vi "Utility Write To Register - Float or Int.vi"(0 "VISA resource name":refnum<visa-resource-name>, 1 "Unit Address (1)":u8=1, 5 "Register Address (0)":u16, 9 "Data (0)":sgl, 11 "error in (no error)":errorcluster) -> (4 "VISA resource name out":refnum<visa-resource-name>, 15 "error out":errorcluster {"code" format="%.0x"})   [LabVIEW 2010, in "Eurotherm 32xx Series.lvlib"]
doc: "This VI writes the value to the specified register of specified unit."
uses:
  <instrlib>/Eurotherm 32xx Series/Eurotherm 32xx Series.lvlib
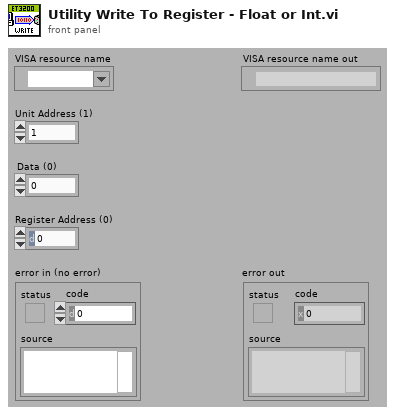
[diagram p1: front panel]
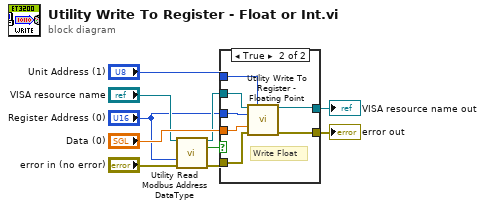
[diagram p0: block diagram]
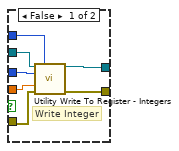
[diagram p2: hidden frame]
diagram:
  n1 = call <instrlib>:"Utility Read Modbus Address DataType.vi"("VISA resource name"="VISA resource name", "Register Address (0)"="Register Address (0)", "error in (no error)"="error in (no error)") -> ("VISA resource name out"=w3:refnum<visa-resource-name>, "Float32 (T)"=w1:bool, "error out"=w5:errorcluster)  [unwired: 9 in, 1 out]
  n2 = case shown="True" w1 {
    tunnel: w3 -> [w17 w22]
    tunnel: "Register Address (0)" -> [w16 w19]
    tunnel: "Data (0)" -> [w15 w20]
    tunnel: w5 -> [w14 w21]
    tunnel: [w13 w24] -> w9
    tunnel: [w12 w23] -> w8
    tunnel: "Unit Address (1)" -> [w11 w18]
    frame False {
      # "Write Integer"
      n3 = call <instrlib>:"Utility Write To Register - Integers.vi"("VISA resource name"=w17, "Unit Address (1)"=w11, "Register Address (0)"=w16, "Data (0)"=w15, "error in (no error)"=w14) -> ("VISA resource name out"=w13:refnum<visa-resource-name>, "error out"=w12:errorcluster)  [unwired: 9 in]
    }
    frame True {
      # "Write Float"
      n4 = call <instrlib>:"Utility Write To Register - Floating Point.vi"("VISA resource name"=w22, "Unit Address (1)"=w18, "Register Address (0)"=w19, "Data (0)"=w20, "error in (no error)"=w21) -> ("VISA resource name out"=w24:refnum<visa-resource-name>, "error out"=w23:errorcluster)  [unwired: 9 in]
    }
  }
  "VISA resource name out" <- w9
  "error out" <- w8
